vi "Get Domain.vi"(8 "error in (no error)":errorcluster, 11 "Mean Fit in":refnum<class "Mean Fit.lvclass">) -> (0 "error out":errorcluster, 1 "Xmax":dbl, 2 "Xmin":dbl, 3 "Mean Fit out":refnum<class "Mean Fit.lvclass">)   [LabVIEW 2016, in "Mean Fit.lvclass"]
uses:
  Mean Fit.lvclass
  Mean Fit.lvclass/Mean Fit.ctl
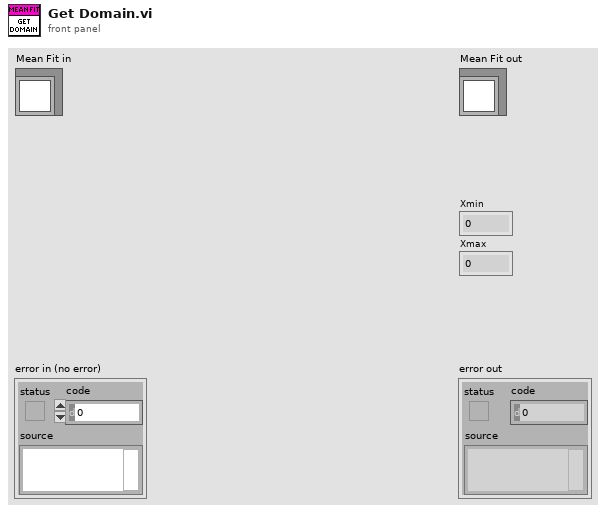
[diagram p1: front panel]
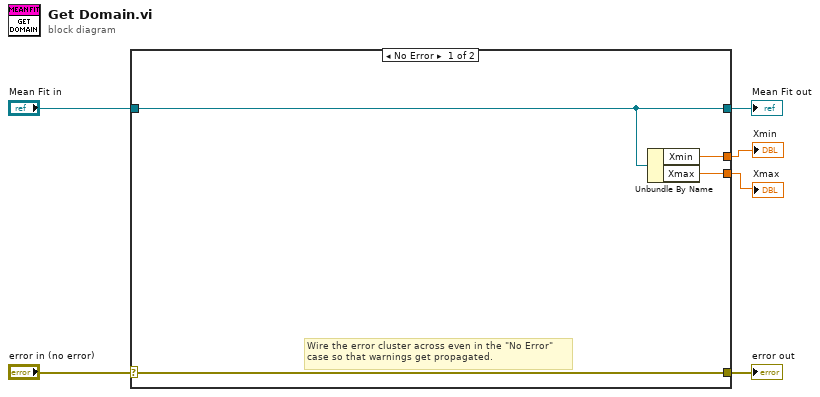
[diagram p0: block diagram]
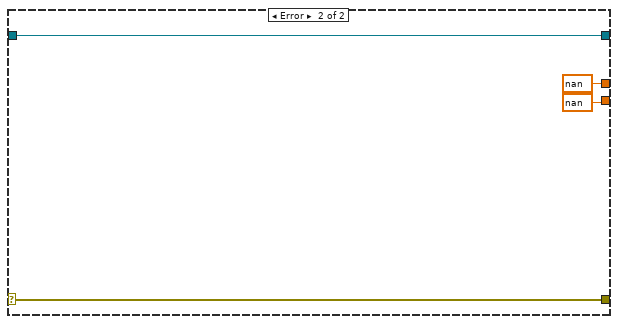
[diagram p2: hidden frame]
diagram:
  n1 = case shown="No Error" "error in (no error)" {
    selector: "error in (no error)" -> [w10 w14]
    tunnel: [w10 w14] -> w5
    tunnel: [w9 w13] -> w3
    tunnel: "Mean Fit in" -> [w9 w13]
    tunnel: [w8 nan ("Xmin")] -> w2
    tunnel: [w7 nan ("Xmax")] -> w1
    frame No Error {
      # "Wire the error cluster across even in the \"No Error\"\ncase so that warnings get propagated."
      n2 = Unbundle By Name(w9) -> ("Xmin"=w8:dbl, "Xmax"=w7:dbl)
    }
    frame Error {
    }
  }
  "error out" <- w5
  "Mean Fit out" <- w3
  "Xmin" <- w2
  "Xmax" <- w1
